vi "recipeScript generatePyScript.vi"(5 "userTable":string[][](array[string]), 7 "instrTable":string[][](array[string]), 8 "error in (no error)":errorcluster, 10 "recipeScript":string, 11 "sourceFilePath":path) -> (0 "error out":errorcluster, 3 "PyCode":string)   [LabVIEW 2018]
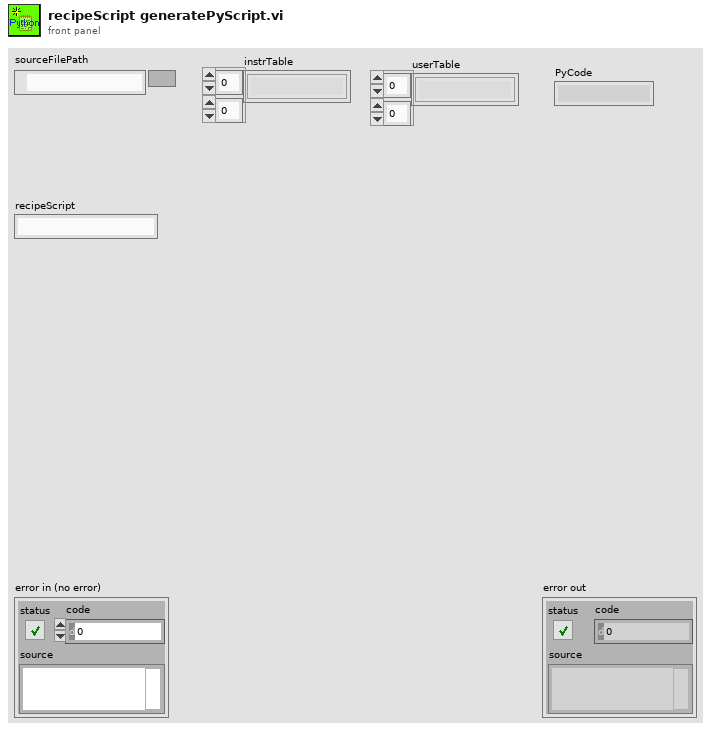
[diagram p1: front panel]
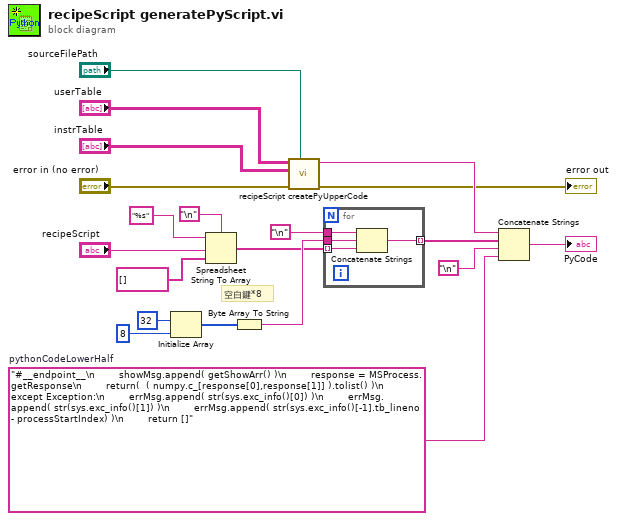
[diagram p0: block diagram]
diagram:
  w4 = "#__endpoint__\n        showMsg.append( getShowArr() )\n        response = MSProcess.getResponse\n        return(  ( numpy.c_[response[0],response[1]] ).tolist() )\n    except Exception:\n        errMsg.append( str(sys.exc_info()[0]) )\n        errMsg.append( str(sys.exc_info()[1]) )\n        errMsg.append( str(sys.exc_info()[-1].tb_lineno - processStartIndex) )\n        return []"  # pythonCodeLowerHalf
  # "空白鍵*8"
  n1 = Initialize Array(u8 32, 8 ("dimension size")) -> (w17:u8[])
  n2 = Spreadsheet String To Array(delimiter (Tab)="\n", format string="%s", spreadsheet string="recipeScript", array type (2D Dbl)=string[] []) -> (array=w9:string[])
  n3 = Byte Array To String(unsigned byte array=w17) -> (string=w16:string)
  n4 = call "recipeScript createPyUpperCode.vi"("filePath"="sourceFilePath", "error in (no error)"="error in (no error)", "instrTable"="instrTable", "userTable"="userTable") -> ("error out"=→"error out":errorcluster, "concatenated string"=w10:string)  [unwired: 6 in]
  n5 = for {
    tunnel: w9 -> [w21] mode=indexing
    tunnel: w16 -> [w24]
    tunnel: [w23] -> w12 mode=indexing
    tunnel: "\n" ("delimiter (Tab)") -> [w22]
    n6 = Concatenate Strings(w22, w24, w21) -> (w23:string)
  }
  n7 = Concatenate Strings(w10, w12, "\n" ("delimiter (Tab)"), w4) -> (→"PyCode":string)
